vi "InitialiseASI_communication.vi"(5 "COM port":refnum<visa-resource-name>="COM17") -> (0 "error out":errorcluster, 2 "VISA resource name out":refnum<visa-resource-name>)   [LabVIEW 2018]
uses:
  <vilib>/Instr/_visa.llb/VISA Configure Serial Port (Instr).vi
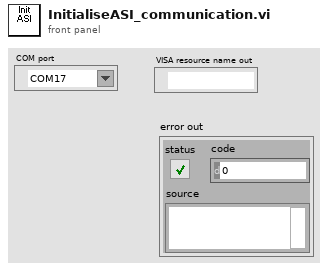
[diagram p1: front panel]
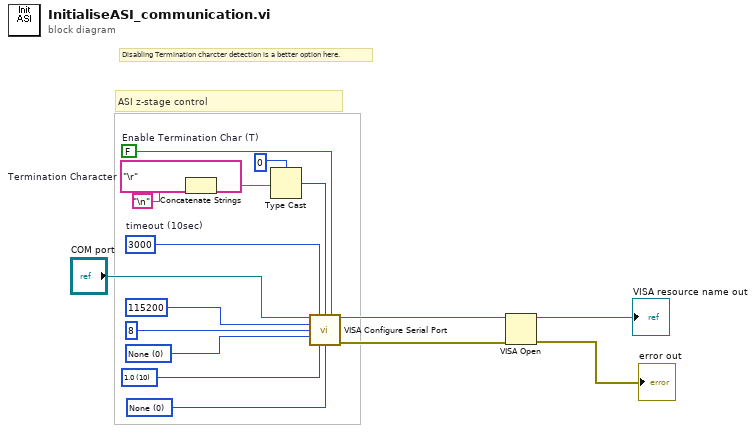
[diagram p0: block diagram]
diagram:
  w4 = u16 0 items=["None"=0, "XON/XOFF"=1, "RTS/CTS"=2, "DTR/DSR"=4] ("flow control")
  w14 = u16 10 items=["1.0"=10, "1.5"=15, "2.0"=20] ("stop bits")
  w11 = u16 0 items=["None", "Odd", "Even", "Mark", "Space"] ("parity")
  w8 = "\r"  # Termination Character
  w13 = FALSE  # Enable Termination Char (T)
  w12 = u32 3000  # timeout (10sec)
  # "Disabling Termination charcter detection is a better option here."
  # "ASI z-stage control"
  n1 = Concatenate Strings(w8, "\n") -> (w6:string)
  n2 = Type Cast(type=u8 0, x=w6) -> (*(type *) &x=w17:u8)
  n3 = call-poly "VISA Configure Serial Port"("VISA resource name"="COM port", "timeout (10sec)"=w12, "termination char\n(0xA = '\\n' = LF)"=w17, "Enable Termination\nChar (T)"=w13, "baud rate (9600)"=u32 115200 ("baud rate"), "data bits (8)"=u16 8 ("data bits"), "parity (0:none)"=w11, "stop bits (10: 1 bit)"=w14, "flow control (0:none)"=w4) -> ("VISA resource name out"=w5:refnum<visa-resource-name>, "error out"=w2:errorcluster)  [unwired: 5 in]
  n4 = VISA Open(error in (no error)=w2, VISA resource name=w5) -> (VISA resource name=→"VISA resource name out":refnum<visa-resource-name>, error out=→"error out":errorcluster)  [unwired: 3 in]
